vi "Teleop.vi"(10 "Match Info":T1={"Autonomous Elapsed Seconds"=0.0, "TeleOp Elapsed Seconds"=0.0, "Disabled Elapsed Seconds"=0.0, "Visited Autonomous"=FALSE, "Visited TeleOp"=FALSE, "Visited Disabled"=FALSE, "Autonomous Settings"={"Autonomous Style"=enum."Independent", "VI Refnum"=refnum}}, 11 "Call Context":T2) -> ()   [LabVIEW 2014]
doc: "This VI is called for each TeleOp packet received from the DS where the robot is not disabled. It is often used to read from the joysticks and update I/O or to update setpoints for timed control loops. It should complete and return within 20 milliseconds or it may miss DS packets."
uses:
  <vilib>/Rock Robotics/WPI/DriverStation/WPI_DriverStationDerivedRobotMode.ctl
  <vilib>/Rock Robotics/WPI/DriverStation/WPI_DriverStationMatch Info.ctl
  DriverButtons.ctl
  OpAxis.ctl
  OpButtons.ctl
  DriverAxis.ctl
  Global Ref.vi
  Robot Values.vi
  DriveGlobal.vi
  Robot Fail.vi
  <vilib>/Rock Robotics/Network Tables/SD Write Numeric Array.vi
  <vilib>/Rock Robotics/Network Tables/SD Read Boolean.vi
  <vilib>/Rock Robotics/Network Tables/SD Write Boolean Array.vi
  <vilib>/Rock Robotics/Network Tables/SD Read Number.vi
panel:
  out "Sample Slider 0":dbl(slide) scale=0.0..5.0
  out "Sample Boolean 1":bool
  out "Sample Boolean 0":bool
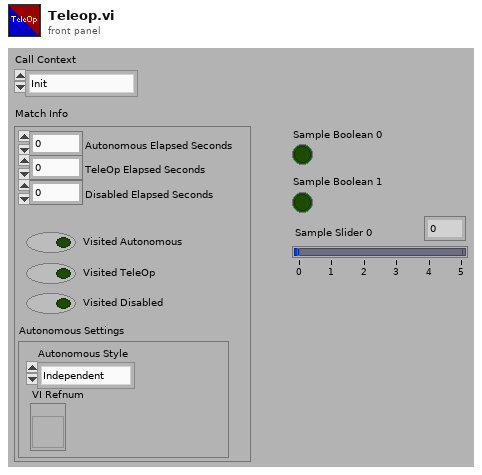
[diagram p1: front panel]
types:
  T1 = typedef "WPI_DriverStationMatch Info.ctl" = cluster{"Autonomous Elapsed Seconds":dbl, "TeleOp Elapsed Seconds":dbl, "Disabled Elapsed Seconds":dbl, "Visited Autonomous":bool, "Visited TeleOp":bool, "Visited Disabled":bool, "Autonomous Settings":cluster{"Autonomous Style":enum16{"Iterative", "Independent"}, "VI Refnum":refnum<vi>}}
  T2 = typedef "WPI_DriverStationDerivedRobotMode.ctl" = enum16{"Init", "Execute", "Stop"}
  T3 = typedef "OpButtons.ctl" = cluster{"Lift Pos 1":bool, "Lift Pos 2":bool, "Lift Pos 3":bool, "Lift Pos 4":bool, "Left Bumper":bool, "Right Bumper":bool, "Boolean 7":bool, "Boolean 8":bool, "Boolean9":bool, "Lift override":bool, "Boolean 11":bool, "Boolean 12":bool}
  T4 = typedef "OpAxis.ctl" = cluster{"Left X":dbl, "Left Y":dbl, "Right X":dbl, "Right Y":dbl, "D-Pad X":dbl, "D-Pad Y":dbl}
  T5 = typedef "DriverButtons.ctl" = cluster{"ToteAutokeep":bool, "ToteAutoSpit":bool, "Boolean 3":bool, "TrackTote":bool, "ToteLeftspit":bool, "ToteRigthspit":bool, "ToteLeftPull":bool, "Control power":bool, "Drive mode":bool, "Boolean 10":bool, "Boolean 11":bool, "ToteRightPull":bool}
  T6 = typedef "DriverAxis.ctl" = cluster{"Left X":dbl, "Left Y":dbl, "Right X":dbl, "Right Y":dbl, "D-Pad X":dbl, "D-Pad Y":dbl}
  T7 = cluster{"Left X":dbl, "Left Y":dbl, "Trigger L":dbl, "Trigger R":dbl, "Right X":dbl, "Right Y":dbl}
  T8 = typedef "WPI_RobotDriveDevRef.ctl" = cluster{"DevStatus":errorcluster, "Motors[]":T9[], "Square Inputs":bool, "Max Output":dbl}
  T9 = typedef "WPI_MotorControlDeviceRef.ctl" = cluster{"DeviceStatus":errorcluster, "Type":T10, "PWM":cluster{"Controller":T11, "PWM Channel":T12, "DeadBand":T13}, "CAN":cluster{"Device Number":u8, "Control Mode":T14, "Semaphore":T15, "Max Vout":dbl, "TalonSRX Control Mode":T16}, "Invert":bool, "TransformRef":T17, "InvTransformRef":T17}
  T10 = typedef "WPI_MotorControlType.ctl" = enum16{"PWM", "CAN", "CANTalonSRX"}
  T11 = typedef "FPGA_TypedefDigitalModule.ctl" = enum16{"Controller 1"}
  T12 = typedef "FPGA_DIOPWMChannel.ctl" = enum8{"PWM 0", "PWM 1", "PWM 2", "PWM 3", "PWM 4", "PWM 5", "PWM 6", "PWM 7", "PWM 8", "PWM 9", "PWM MXP 0", "PWM MXP 1", "PWM MXP 2", "PWM MXP 3", "PWM MXP 4", "PWM MXP 5", "PWM MXP 6", "PWM MXP 7", "PWM MXP 8", "PWM MXP 9", "Invalid"}
  T13 = typedef "WPI_PWMDeadband.ctl" = cluster{"Name":string, "maxPositivePwm":i32, "minPositivePwm":i32, "centerPwm":i32, "maxNegativePwm":i32, "minNegativePwm":i32, "angularRange":u16}
  T14 = typedef "WPI_CANJaguar_ControlMode.ctl" = enum8{"Percent VBus", "Current", "Speed", "Position", "Voltage"}
  T15 = typedef "Semaphore RefNum" = refnum<k1>
  T16 = typedef "WPI_CANTalonSRX_APIControlMode.ctl" = enum8{"Percent VBus", "Speed", "Position", "Slave", "Unchanged / Invalid"}
  T17 = typedef "WPI_PWMTransform_ConPane.ctl" = refnum<vi>
  T18 = typedef "WPI_JoystickDevRef.ctl" = cluster{"Device":T19}
  T19 = typedef "WPI_JoystickDeviceEnum.ctl" = enum16{"USB 0", "USB 1", "USB 2", "USB 3", "USB 4", "USB 5"}
  T20 = typedef "Global Ref typedef.ctl" = cluster{"Drive":cluster{"RobotDriveDevRef":T8}, "Joysticks":cluster{"JoyDriveRef":T18, "JoyOpRef":T18, "JoySabatourRef":T18}, "Lift":cluster{"LiftMotorRefLeft":T9, "LiftMotorRefRight":T9}, "Lift Limits":cluster{"Bottom Left":T21, "Bottom Right":T21}, "Accel":cluster{"AccelerometerDevRef":T23}, "Lift Encoder":cluster{"AIDeviceRefRight":T32, "AIDeviceRefLeft":T32}, "Lights":cluster{"Swag Light Ref cluster":cluster{"PWMDeviceRef1":T33, "PWMDeviceRef2":T33, "PWMDeviceRef3":T33, "PWMDeviceRef4":T33, "PWMDeviceRef5":T33, "PWMDeviceRef6":T33, "PWMDeviceRef7":T33, "PWMDeviceRef8":T33}}, "Camera":cluster{"GrayScaleImage":T34, "ColorImage":T34, "CameraDevRef":T35}, "Drive Encoders":cluster{"AIDeviceRef Left":T32, "AIDeviceRef Right":T32}, "Gyro":cluster{"GyroDevRef":T36}, "Relay":cluster{"RelayDevRef":T37, "RelayDevRef 2":T37}}
  T21 = typedef "WPI_DigitalInputDevRef.ctl" = cluster{"DevStatus":errorcluster, "DIO Channel":T22, "Controller":T11}
  T22 = typedef "FPGA_DIOChannel.ctl" = enum8{"DIO 0", "DIO 1", "DIO 2", "DIO 3", "DIO 4", "DIO 5", "DIO 6", "DIO 7", "DIO 8", "DIO 9", "DIO MXP 0", "DIO MXP 1", "DIO MXP 2", "DIO MXP 3", "DIO MXP 4", "DIO MXP 5", "DIO MXP 6", "DIO MXP 7", "DIO MXP 8", "DIO MXP 9", "DIO MXP 10", "DIO MXP 11", "DIO MXP 12", "DIO MXP 13", "DIO MXP 14", "DIO MXP 15", "Invalid"}
  T23 = typedef "WPI_AccelerometerDevRef.ctl" = cluster{"DevStatus":errorcluster, "Controller":T24, "Scaling":T25, "Analog Channels":T26, "I2C Bus":T28, "SPI Bus":T29, "Accel Range":T30, "ADXL345 Axes":T31, "Handle":i32, "Device Address":u8, "Accel Type":enum16{"Analog", "ADXL345 I2C", "ADXL345 SPI", "Internal"}}
  T24 = typedef "FPGA_TypedefAnalogModule.ctl" = enum16{"Controller 1"}
  T25 = typedef "WPI_AccelerometerScaling.ctl" = cluster{"Gain (VoltsPerG)":dbl, "Center Voltage":dbl}
  T26 = typedef "WPI_AccelerometerAnalogChannels.ctl" = cluster{"X-Axis":T27, "Y-Axis":T27, "Z-Axis":T27}
  T27 = typedef "FPGA_AIChannel.ctl" = enum8{"AI 0", "AI 1", "AI 2", "AI 3", "AI MXP 0", "AI MXP 1", "AI MXP 2", "AI MXP 3", "Invalid"}
  T28 = typedef "i2c_bus.ctl" = enum16{"I2C On-Board", "I2C MXP", "Invalid"}
  T29 = typedef "spi_bus.ctl" = enum16{"SPI On-Board, CS0", "SPI On-Board, CS1", "SPI On-Board, CS2", "SPI On-Board, CS3", "SPI MXP", "Invalid"}
  T30 = typedef "ADXL345 Range.ctl" = u8
  T31 = typedef "WPI_AccelerometerADXL345 Axes.ctl" = cluster{"X-Axis":bool, "Y-Axis":bool, "Z-Axis":bool}
  T32 = typedef "WPI_AnalogChannelDevRef.ctl" = cluster{"DevStatus":errorcluster, "Controller":T24, "Analog Channel":T27}
  T33 = typedef "WPI_PWMDeviceRef.ctl" = cluster{"DeviceStatus":errorcluster, "Controller":T11, "PWM Channel":T12}
  T34 = typedef "IMAQ Image.ctl" = refnum<image>
  T35 = typedef "WPI_CameraDevRef.ctl" = cluster{"Camera Address":string, "CameraStatus":errorcluster}
  T36 = typedef "WPI_GyroDevRef.ctl" = cluster{"DevStatus":errorcluster, "Analog Module":T24, "Analog Channel":T27, "Offset":dbl, "Gain (VoltsPerDegree/Second)":dbl}
  T37 = typedef "WPI_RelayDevRef.ctl" = cluster{"DevStatus":errorcluster, "Relay Channel":T38, "Controller":T11, "Relay Direction":T39}
  T38 = typedef "FPGA_DIORelayChannel.ctl" = enum8{"Relay 0", "Relay 1", "Relay 2", "Relay 3", "Invalid"}
  T39 = typedef "WPI_RelayDirection.ctl" = enum16{"Both directions", "Forward only", "Reverse only"}
  T40 = cluster{"DriveMode":enum16{"Tank", "Arcade"}, "Is Logitech":bool}
  T41 = cluster{"Tracking Tote?":bool, "ToteRightSpeed":dbl, "ToteLeftSpeed":dbl, "Drive Encoder reset":bool, "Right Wheel \n(Cm)":dbl, "Left Wheel \n(Cm)":dbl}
  T42 = cluster{"Lift Position":i32, "Lift Speed Override":dbl, "OverrideTele?":bool, "OverrideDash":bool}
  T43 = cluster{"RightMotorSpeed":dbl, "LeftMotorSpeed":dbl}
  T44 = cluster{"Not stright - Right":bool, "Not stright - Left":bool, "Lift position change":bool, "Lift out of sync":bool, "Joystick sensitivity Less":bool, "Stuck in Tank":bool, "Joystick Sensistiviy More":bool}
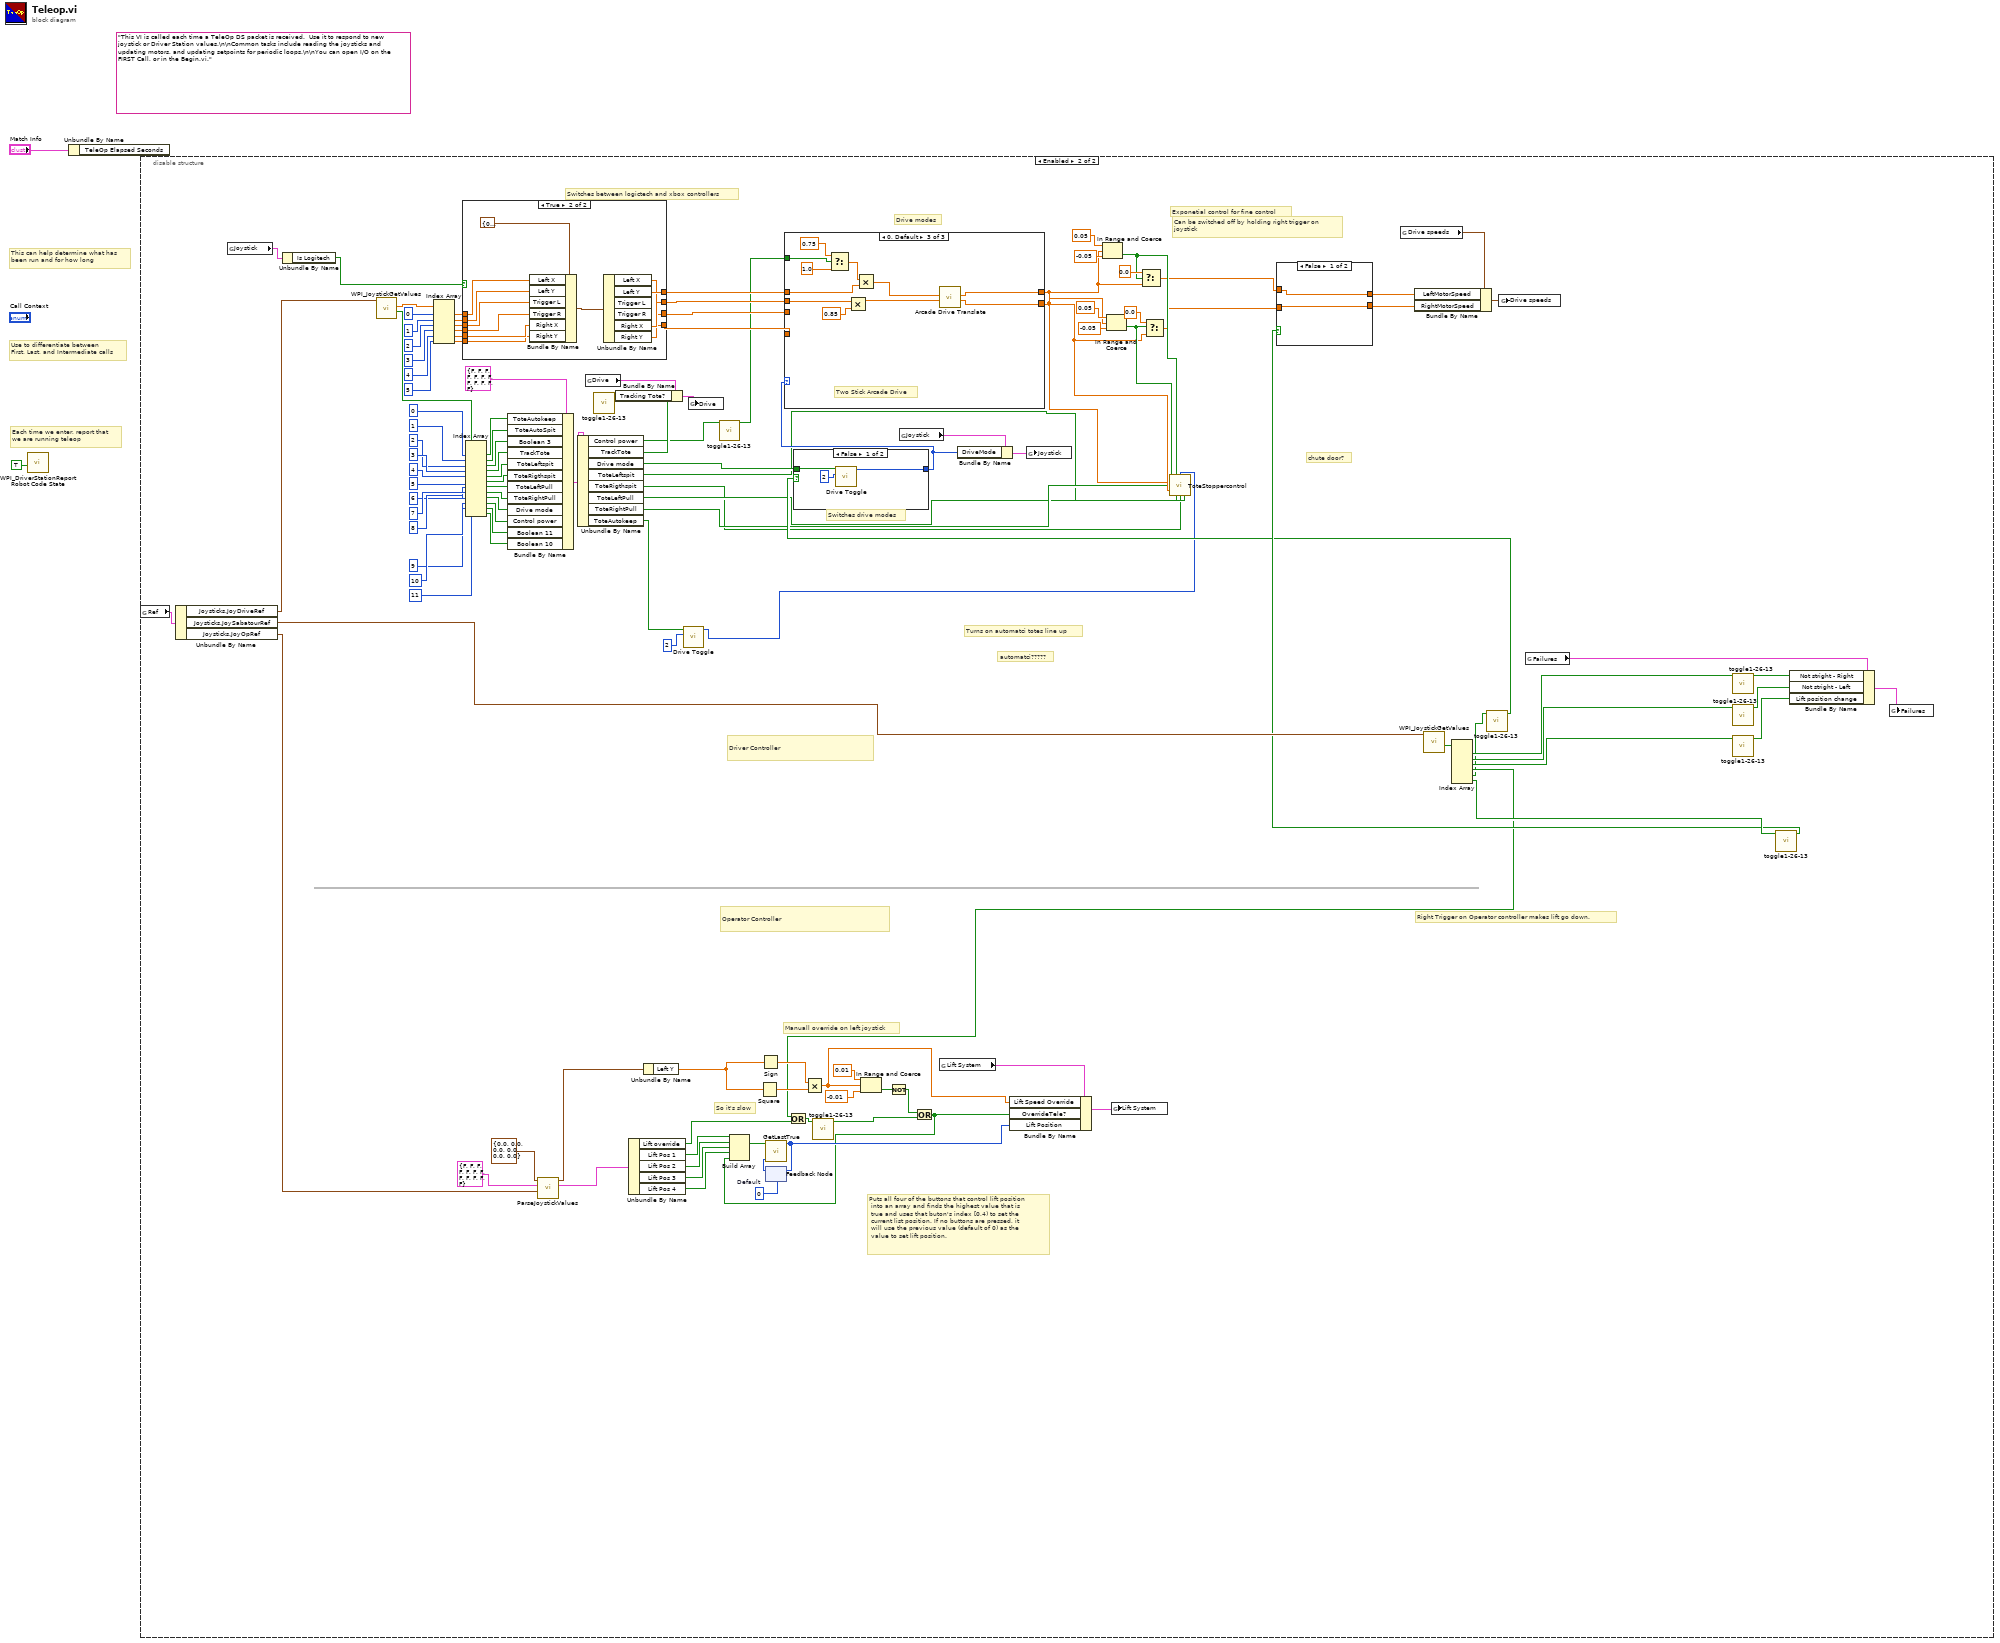
[diagram p0: block diagram]
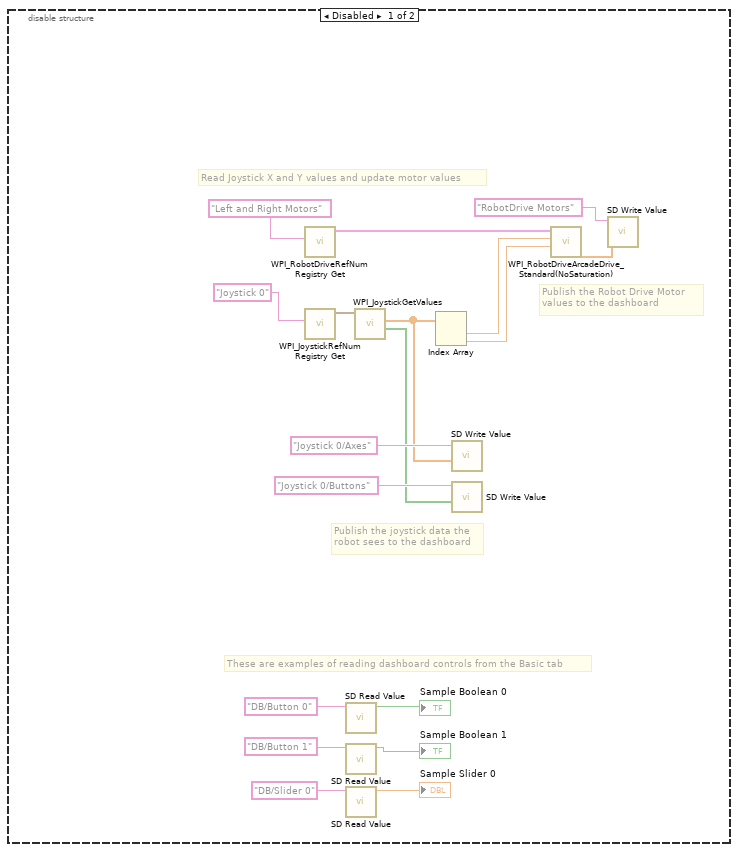
[diagram p2: hidden frame]
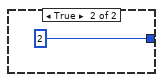
[diagram p3: hidden frame]
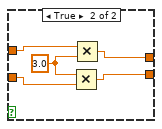
[diagram p4: hidden frame]
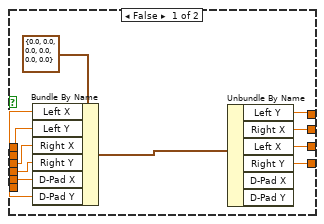
[diagram p5: hidden frame]
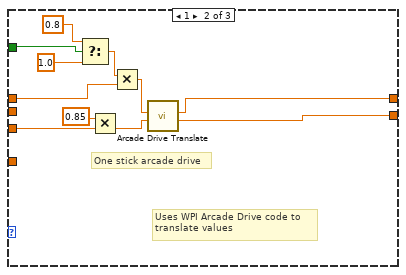
[diagram p7: hidden frame]
diagram:
  (unwired) "This VI is called each time a TeleOp DS packet is received.  Use it to respond to new joystick or Driver Station values.\n\nCommon tasks include reading the joysticks and updating motors, and updating setpoints for periodic loops.\n\nYou can open I/O on the FIRST Call, or in the Begin.vi."
  # "Each time we enter, report that\nwe are running teleop"
  # "Use to differentiate between\nFirst, Last, and Intermediate calls"
  # "This can help determine what has\nbeen run and for how long"
  n1 = call <vilib>:"WPI_DriverStationReport Robot Code State.vi"("TeleOp"=TRUE ("Autonomous")) -> ()  [unwired: 10 in, 1 out]
  n2 = Unbundle By Name("Match Info") -> ()  [unwired: 1 out]
  n3 = disable-structure shown="Enabled" {
    frame Disabled {
      # "These are examples of reading dashboard controls from the Basic tab"
      # "Publish the Robot Drive Motor\nvalues to the dashboard"
      # "Publish the joystick data the\nrobot sees to the dashboard"
      # "Read Joystick X and Y values and update motor values"
      n4 = call <vilib>:"WPI_RobotDriveRefNum Registry Get.vi"("refnum name"="Left and Right Motors") -> ("RobotDriveDevRef"=w19:T8)  [unwired: 1 in, 9 out]
      n5 = call <vilib>:"WPI_JoystickRefNum Registry Get.vi"("refnum name"="Joystick 0") -> ("JoystickDevRef"=w16:T18)  [unwired: 1 in, 9 out]
      n6 = call-poly <vilib>:"SD Read Value.vi"("Name"="DB/Button 0" ("refnum name")) -> ("Boolean"=→"Sample Boolean 0":bool)  [unwired: 8 in, 2 out]
      n7 = call-poly <vilib>:"SD Read Value.vi"("Name"="DB/Button 1" ("refnum name")) -> ("Boolean"=→"Sample Boolean 1":bool)  [unwired: 8 in, 2 out]
      n8 = call-poly <vilib>:"SD Read Value.vi"("Name"="DB/Slider 0" ("refnum name")) -> ("Numeric"=→"Sample Slider 0":dbl)  [unwired: 8 in, 2 out]
      n9 = call <vilib>:"WPI_JoystickGetValues.vi"("JoystickDevRef"=w16) -> ("Buttons"=w3:bool[], "Axes"=w5:dbl[])  [unwired: 6 in, 3 out]
      n10 = Index Array(array=w5) -> (element #1=w18:dbl, element #2=w8:dbl)  [unwired: 2 in]
      n11 = call-poly <vilib>:"SD Write Value.vi"("Numeric Array"=w5, "Name"="Joystick 0/Axes") -> ()  [unwired: 8 in, 2 out]
      n12 = call-poly <vilib>:"SD Write Value.vi"("Boolean Array"=w3, "Name"="Joystick 0/Buttons") -> ()  [unwired: 8 in, 2 out]
      n13 = call <vilib>:"WPI_RobotDriveArcadeDrive_Standard(NoSaturation).vi"("Y axis value"=w8, "X axis value"=w18, "RobotDriveDevRef"=w19) -> ("Motor Values"=w7:dbl[])  [unwired: 1 in, 7 out]
      n14 = call-poly <vilib>:"SD Write Value.vi"("Numeric Array"=w7, "Name"="RobotDrive Motors") -> ()  [unwired: 8 in, 2 out]
    }
    frame Enabled {
      w83 = 0  # Default
      # "chute door?"
      # "automatci?????"
      # "Right Trigger on Operator controller makes lift go down."
      # "Manuall override on left joystick"
      # "Switches drive modes"
      # "Turns on automatci totes line up"
      # "Can be switched off by holding right trigger on \njoystick"
      # "Exponetial control for fine control"
      # "Drive modes"
      # "Switches between logictech and xbox controllers"
      # "So it's slow"
      # "Puts all four of the buttons that control lift position\n into an array and finds the highest value that is \n true and uses that buton's index [0,4) to set the\n current list position. If no buttons are pressed, it\n will use the previous value (default of 0) as the\n value to set lift position."
      # "Driver Controller"
      # "Operator Controller"
      n15 = global read "Global Ref.vi" "Ref"() -> (w143:T20)
      n16 = Unbundle By Name(w143) -> ("Joysticks.JoyDriveRef"=w87:T18, "Joysticks.JoySabatourRef"=w54:T18, "Joysticks.JoyOpRef"=w139:T18)
      n17 = global read "Robot Values.vi" "Joystick"() -> (w73:T40)
      n18 = Unbundle By Name(w73) -> ("Is Logitech"=w72:bool)
      n19 = call <vilib>:"WPI_JoystickGetValues.vi"("JoystickDevRef"=w87) -> ("Buttons"=w127:bool[], "Axes"=w101:dbl[])  [unwired: 6 in, 3 out]
      n20 = Index Array(array=w101, index #1=0 ("index"), index #2=1 ("index"), index #3=2 ("index"), index #4=3 ("index"), index #5=4 ("index"), index #6=5 ("index")) -> (element #1=w95:dbl, element #2=w96:dbl, element #3=w97:dbl, element #4=w98:dbl, element #5=w99:dbl, element #6=w100:dbl)
      n21 = case shown="True" w72 {
        tunnel: w100 -> [w166 w172]
        tunnel: w99 -> [w165 w173]
        tunnel: w98 -> [w164 w174]
        tunnel: w97 -> [w163 w175]
        tunnel: w96 -> [w162 w176]
        tunnel: w95 -> [w161 w177]
        tunnel: [w158 w170] -> w77
        tunnel: [w157 w169] -> w76
        tunnel: [w156 w167] -> w75
        tunnel: [w155 w168] -> w74
        frame False {
          n22 = Bundle By Name(cluster=T6 {"Left X"=0.0, "Left Y"=0.0, "Right X"=0.0, "Right Y"=0.0, "D-Pad X"=0.0, "D-Pad Y"=0.0} ("input cluster"), "Left X"=w161, "Left Y"=w162, "Right X"=w163, "Right Y"=w164, "D-Pad X"=w165, "D-Pad Y"=w166) -> (w160:T6)
          n23 = Unbundle By Name(w160) -> ("Left Y"=w158:dbl, "Right X"=w157:dbl, "Left X"=w155:dbl, "Right Y"=w156:dbl)  [unwired: 2 out]
        }
        frame True {
          n24 = Bundle By Name(cluster=T7 {"Left X"=0.0, "Left Y"=0.0, "Trigger L"=0.0, "Trigger R"=0.0, "Right X"=0.0, "Right Y"=0.0} ("Xbox Axis"), "Left X"=w177, "Left Y"=w176, "Trigger L"=w175, "Trigger R"=w174, "Right X"=w173, "Right Y"=w172) -> (w171:T7)
          n25 = Unbundle By Name(w171) -> ("Left X"=w168:dbl, "Left Y"=w170:dbl, "Right X"=w169:dbl, "Right Y"=w167:dbl)  [unwired: 2 out]
        }
      }
      n26 = Index Array(array=w127, index #1=0 ("index"), index #2=1 ("index"), index #3=2 ("index"), index #4=3 ("index"), index #5=4 ("index"), index #6=5 ("index"), index #7=6 ("index"), index #8=7 ("index"), index #9=8 ("index"), index #10=9 ("index"), index #11=10 ("index"), index #12=11 ("index")) -> (element #1=w115:bool, element #2=w116:bool, element #3=w117:bool, element #4=w118:bool, element #5=w119:bool, element #6=w120:bool, element #7=w121:bool, element #8=w122:bool, element #9=w123:bool, element #10=w124:bool, element #11=w125:bool, element #12=w126:bool)
      n27 = Bundle By Name(cluster=T5 {"ToteAutokeep"=FALSE, "ToteAutoSpit"=FALSE, "Boolean 3"=FALSE, "TrackTote"=FALSE, "ToteLeftspit"=FALSE, "ToteRigthspit"=FALSE, "ToteLeftPull"=FALSE, "Control power"=FALSE, "Drive mode"=FALSE, "Boolean 10"=FALSE, "Boolean 11"=FALSE, "ToteRightPull"=FALSE} ("Cluster"), "ToteAutokeep"=w115, "ToteAutoSpit"=w116, "Boolean 3"=w117, "TrackTote"=w118, "ToteLeftspit"=w119, "ToteRigthspit"=w120, "ToteLeftPull"=w121, "ToteRightPull"=w122, "Drive mode"=w123, "Control power"=w124, "Boolean 11"=w125, "Boolean 10"=w126) -> (w89:T5)
      n28 = call "ParseJoystickValues.vi"("JoyRef"=w139, "Button Names"=T3 {"Lift Pos 1"=FALSE, "Lift Pos 2"=FALSE, "Lift Pos 3"=FALSE, "Lift Pos 4"=FALSE, "Left Bumper"=FALSE, "Right Bumper"=FALSE, "Boolean 7"=FALSE, "Boolean 8"=FALSE, "Boolean9"=FALSE, "Lift override"=FALSE, "Boolean 11"=FALSE, "Boolean 12"=FALSE} ("input cluster"), "Axis Names"=T4 {"Left X"=0.0, "Left Y"=0.0, "Right X"=0.0, "Right Y"=0.0, "D-Pad X"=0.0, "D-Pad Y"=0.0} ("input cluster")) -> ("Named Button Values"=w130:T3, "Named Axis Values"=w131:T4)  [unwired: 7 in]
      n29 = Unbundle By Name(w89) -> ("Control power"=w29:bool, "TrackTote"=w81:bool, "Drive mode"=w86:bool, "ToteLeftspit"=w24:bool, "ToteRigthspit"=w25:bool, "ToteLeftPull"=w26:bool, "ToteRightPull"=w27:bool, "ToteAutokeep"=w22:bool)
      n30 = global read "Robot Values.vi" "Drive"() -> (w80:T41)
      n31 = call "toggle1-26-13.vi"("input"=w81) -> ("output"=w78:bool)  [unwired: 10 in]
      n32 = Bundle By Name(cluster=w80, "Tracking Tote?"=w78) -> (w79:T41)
      n33 = Unbundle By Name(w130) -> ("Lift override"=w62:bool, "Lift Pos 1"=w138:bool, "Lift Pos 2"=w137:bool, "Lift Pos 3"=w136:bool, "Lift Pos 4"=w135:bool)
      n34 = Unbundle By Name(w131) -> ("Left Y"=w71:dbl)
      n35 = call "Drive Toggle.vi"("Limit"=2, "Button"=w22) -> ("Output"=w23:i32)  [unwired: 9 in]
      n36 = global write "Robot Values.vi" "Drive"(w79) -> ()
      n37 = call "toggle1-26-13.vi"("input"=w29) -> ("output"=w28:bool)  [unwired: 10 in]
      n38 = Square(x=w71) -> (x^2=w82:dbl)
      n39 = Sign(1:w71) -> (0:w70:dbl)
      n40 = feedback #1(w83) -> (w84:i32)
      n41 = Multiply(x=w70, y=w82) -> (x*y=w67:dbl)
      n42 = In Range and Coerce(upper limit=0.01, x=w67, lower limit=-0.01) -> (In Range?=w66:bool)  [unwired: 1 out]
      n43 = Not(x=w66) -> (.not. x?=w65:bool)
      n44 = global read "Robot Values.vi" "Joystick"() -> (w142:T40)
      n45 = global read "Robot Values.vi" "Lift System"() -> (w133:T42)
      n46 = global read "DriveGlobal.vi" "Drive speeds"() -> (w63:T43)
      n47 = call <vilib>:"WPI_JoystickGetValues.vi"("JoystickDevRef"=w54) -> ("Buttons"=w53:bool[])  [unwired: 6 in, 4 out]
      n48 = Index Array(array=w53) -> (element #1=w50:bool, element #2=w49:bool, element #3=w48:bool, element #4=w39:bool, element #5=w38:bool, element #6=w42:bool)  [unwired: 6 in]
      n49 = Or(x=w39, y=w62) -> (x .or. y?=w40:bool)
      n50 = call "toggle1-26-13.vi"("input"=w40) -> ("output"=w61:bool)  [unwired: 10 in]
      n51 = Or(x=w65, y=w61) -> (x .or. y?=w32:bool)
      n52 = Build Array(w138, w137, w136, w135, w32) -> (w85:bool[])
      n53 = call "GetLastTrue.vi"("Default value"=w84, "Input"=w85) -> ("Last True"=w132:i32)  [unwired: 9 in]
      n54 = feedback-in #1(w132) -> ()
      n55 = Bundle By Name(cluster=w133, "Lift Speed Override"=w67, "OverrideTele?"=w32, "Lift Position"=w132) -> (w134:T42)
      n56 = global write "Robot Values.vi" "Lift System"(w134) -> ()
      n57 = call "toggle1-26-13.vi"("input"=w38) -> ("output"=w37:bool)  [unwired: 10 in]
      n58 = case shown="False" w37 {
        tunnel: [w145 2 ("Output")] -> w140
        tunnel: w86 -> [w144 _]
        frame False {
          n59 = call "Drive Toggle.vi"("Limit"=2, "Button"=w144) -> ("Output"=w145:i32)  [unwired: 9 in]
        }
        frame True {
        }
      }
      n60 = case shown="0, Default" w140 {
        tunnel: w77 -> [w180 w186 w197]
        tunnel: w76 -> [_ _ w200]
        tunnel: w75 -> [w179 _ _]
        tunnel: w74 -> [_ w189 _]
        tunnel: [w180 w191 w202] -> w33
        tunnel: [w179 w190 w201] -> w34
        tunnel: w28 -> [_ w181 w192]
        frame 2 {
          # "This is Tank Drive"
          # "Gets joystick values and saves\nthem to the Robot Values typedef"
        }
        frame 1 {
          # "One stick arcade drive"
          # "Uses WPI Arcade Drive code to\ntranslate values"
          n61 = Select(t=0.8, s=w181, f=1.0 ("x")) -> (s? t:f=w182:dbl)
          n62 = Multiply(x=0.85, y=w189) -> (x*y=w188:dbl)
          n63 = Multiply(x=w182, y=w186) -> (x*y=w185:dbl)
          n64 = call "Arcade Drive Translate.vi"("xAxis"=w188, "yAxis"=w185) -> ("outputX"=w190:dbl, "outputY"=w191:dbl)  [unwired: 7 in]
        }
        frame 0, Default {
          # "Two Stick Arcade Drive"
          n65 = Select(t=0.75, s=w192, f=1.0 ("x")) -> (s? t:f=w194:dbl)
          n66 = Multiply(x=w200, y=0.85) -> (x*y=w199:dbl)
          n67 = Multiply(x=w194, y=w197) -> (x*y=w196:dbl)
          n68 = call "Arcade Drive Translate.vi"("xAxis"=w199, "yAxis"=w196) -> ("outputX"=w201:dbl, "outputY"=w202:dbl)  [unwired: 7 in]
        }
      }
      n69 = Bundle By Name(cluster=w142, "DriveMode"=w140) -> (w141:T40)
      n70 = global write "Robot Values.vi" "Joystick"(w141) -> ()
      n71 = In Range and Coerce(upper limit=0.05, x=w33, lower limit=-0.05) -> (In Range?=w36:bool)  [unwired: 1 out]
      n72 = In Range and Coerce(upper limit=0.05, x=w34, lower limit=-0.05) -> (In Range?=w35:bool)  [unwired: 1 out]
      n73 = Select(t=0.0, s=w36, f=w33) -> (s? t:f=w31:dbl)
      n74 = Select(t=0.0, s=w35, f=w34) -> (s? t:f=w30:dbl)
      n75 = call "ToteStoppercontrol.vi"("Right moving"=w35, "Left moving?"=w36, "Last True"=w23, "outputY"=w33, "ToteRightPull"=w27, "outputX"=w34, "ToteLeftspit"=w24, "ToteRigthspit"=w25, "ToteLeftPull"=w26) -> ()  [unwired: 7 in]
      n76 = global read "Robot Fail.vi" "Failures"() -> (w51:T44)
      n77 = call "toggle1-26-13.vi"("input"=w50) -> ("output"=w47:bool)  [unwired: 10 in]
      n78 = call "toggle1-26-13.vi"("input"=w49) -> ("output"=w46:bool)  [unwired: 10 in]
      n79 = call "toggle1-26-13.vi"("input"=w48) -> ("output"=w45:bool)  [unwired: 10 in]
      n80 = call "toggle1-26-13.vi"("input"=w42) -> ("output"=w41:bool)  [unwired: 10 in]
      n81 = case shown="False" w41 {
        tunnel: w31 -> [w149 w153]
        tunnel: w30 -> [w148 w154]
        tunnel: [w149 w152] -> w44
        tunnel: [w148 w151] -> w43
        frame False {
        }
        frame True {
          w150 = 3.0
          n82 = Multiply(x=w150, y=w154) -> (x*y=w151:dbl)
          n83 = Multiply(x=w153, y=w150) -> (x*y=w152:dbl)
        }
      }
      n84 = Bundle By Name(cluster=w63, "LeftMotorSpeed"=w44, "RightMotorSpeed"=w43) -> (w64:T43)
      n85 = global write "DriveGlobal.vi" "Drive speeds"(w64) -> ()
      n86 = Bundle By Name(cluster=w51, "Not stright - Right"=w47, "Not stright - Left"=w46, "Lift position change"=w45) -> (w52:T44)
      n87 = global write "Robot Fail.vi" "Failures"(w52) -> ()
    }
  }
